vi "FT_Status to Error.vi"(8 "error in (no error)":errorcluster, 10 "FT_Status":u32) -> (0 "error out":errorcluster)   [LabVIEW 2019, in "D2XX-lv.lvlib"]
doc: "Convert FT_STAUS to LabVIEW error"
uses:
  D2XX-lv.lvlib
  <instrlib>/_D2XX/D2XX/D2XX.lvlib
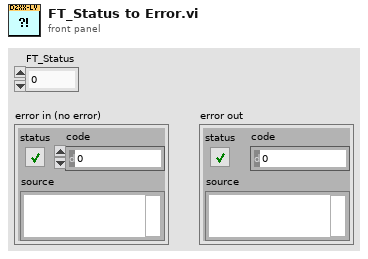
[diagram p1: front panel]
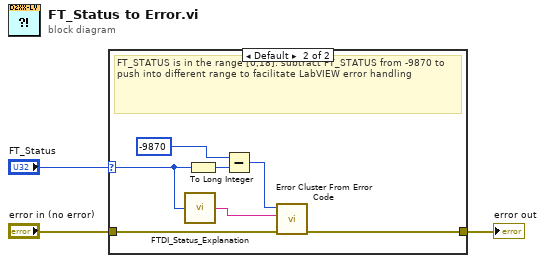
[diagram p0: block diagram]
diagram:
  n1 = case shown="Default" "FT_Status" {
    selector: "FT_Status" -> [_ w9]
    tunnel: "error in (no error)" -> [w4 w11]
    tunnel: [w4 w6] -> w2
    frame 0 {
      # "FT_OK = 0"
    }
    frame Default {
      # "FT_STATUS is in the range [0,18]: subtract FT_STATUS from -9870 to push into different range to facilitate LabVIEW error handling"
      n2 = call <instrlib>:"FTDI_Status_Explanation.vi"("FT_Status"=w9) -> ("Status String"=w10:string)
      n3 = To Long Integer(number=w9) -> (32bit integer=w7:i32)
      n4 = Subtract(x=-9870, y=w7) -> (x-y=w5:i32)
      n5 = call <vilib>:"Error Cluster From Error Code.vi"("error in (no error)"=w11, "error message (\"\")"=w10, "error code (0)"=w5) -> ("error out"=w6:errorcluster)  [unwired: 6 in]
    }
  }
  "error out" <- w2
